vi "Draw.vi"(8 "error in (no error)":errorcluster, 9 "disable contained items?":bool, 10 "IB_SourceTree in":refnum<class "IB_Tree.lvclass">, 11 "IB_TreeMyComputer in":refnum<class "IB_Tree_Item_Proj_MyComputer.lvclass">) -> (0 "error out":errorcluster, 3 "IB_TreeItem out":refnum<class "IB_Tree_Item_Proj_MyComputer.lvclass">)   [LabVIEW 2020, in "IB_Tree_Item_Proj_MyComputer.lvclass"]
uses:
  <vilib>/AppBuilder/IB_Classes/Tree_Item_Proj_MyComputer/IB_Tree_Item_Proj_MyComputer.lvclass
  <vilib>/AppBuilder/IB_Classes/Tree_Item_Proj_MyComputer/IB_Tree_Item_Proj_MyComputer.lvclass/IB_Tree_Item_Proj_MyComputer.ctl
  <resource>/Framework/Providers/Builds/Installer/controls/IB_Tree_DefaultSymbols.ctl
  <vilib>/AppBuilder/IB_Classes/Tree_Source/IB_Tree_Source.lvclass
  <vilib>/AppBuilder/IB_Classes/Tree/IB_Tree.lvclass
  <vilib>/AppBuilder/IB_Classes/Tree_Item/IB_Tree_Item.lvclass
  <vilib>/AppBuilder/IB_Classes/Tree_Item_Proj/IB_Tree_Item_Proj.lvclass
  e:/builds/penguin/labview/branches/2020/dev/dist/vi.lib/AppBuilder/IB_Classes/Tree_Item_Proj_Container/IB_Tree_Item_Proj_Container.lvclass
  e:/builds/penguin/labview/branches/2020/dev/dist/vi.lib/AppBuilder/IB_Classes/Tree_Item_Proj/IB_Tree_Item_Proj.lvclass
  e:/builds/penguin/labview/branches/2020/dev/dist/vi.lib/AppBuilder/IB_Classes/Tree_Item/IB_Tree_Item.lvclass
  e:/builds/penguin/labview/branches/2020/dev/dist/vi.lib/AppBuilder/IB_Classes/Tree_Item_Proj_MyComputer/IB_Tree_Item_Proj_MyComputer.lvclass
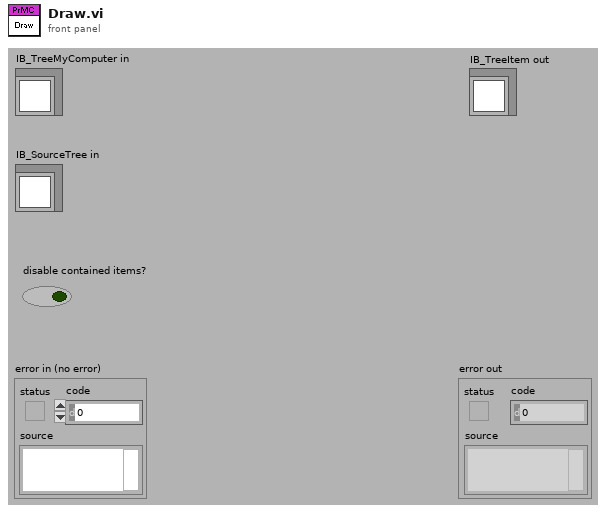
[diagram p1: front panel]
types:
  T1 = typedef "IB_Tree_DefaultSymbols.ctl" = enum16{"<unknown>", "closed folder", "open folder", "closed folder (default)", "open folder (default)", "closed sync folder", "open sync folder", "container folder", "my computer", "build specs", "exe", "dll", "source dist", "restful web service", ".net", "packed library", "c-generator", "target"}
  T2 = typedef "IB_Tree_Source.ctl" = cluster{"buildObject":T3}
  T3 = typedef "ItemRef.ctl" = u64
  T4 = typedef "IB_Tree_Item_Proj.ctl" = cluster{"itemID":string, "path":path}
  T5 = typedef "IB_Tree_Item.ctl" = cluster{"symbol index":i32, "child tag":string, "parentTag":string, "left cell name":string}
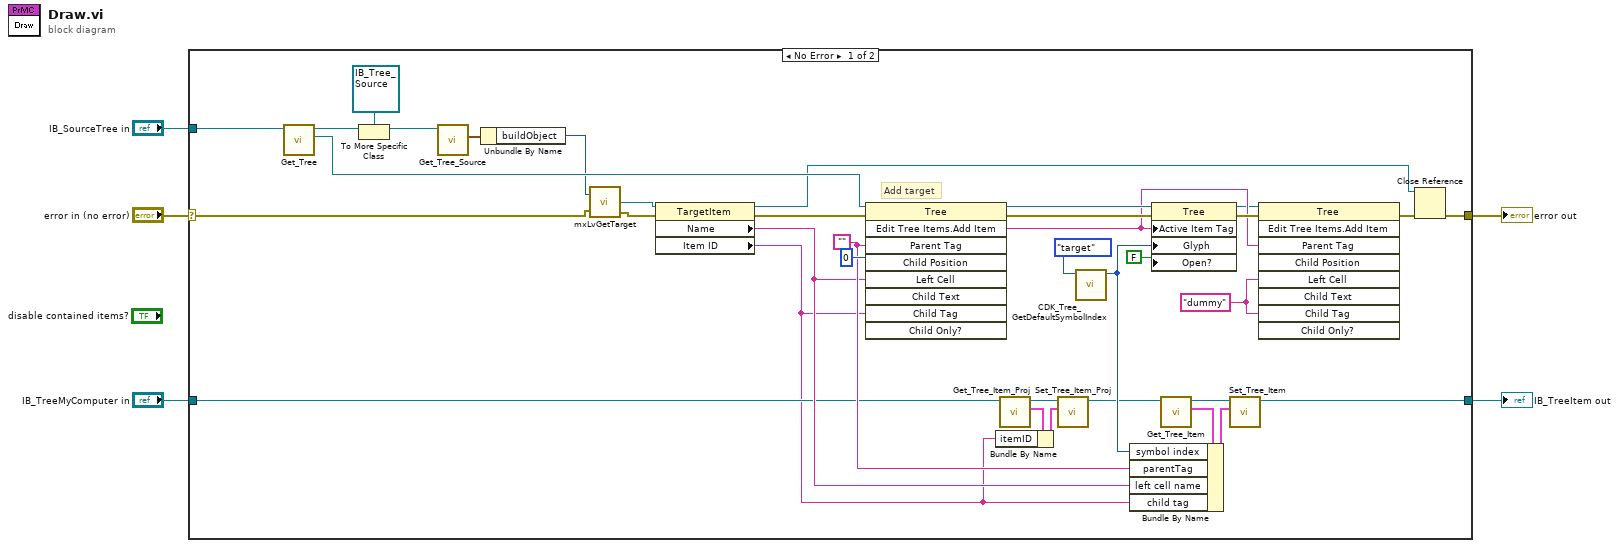
[diagram p0: block diagram]
diagram:
  n1 = case shown="No Error" "error in (no error)" {
    selector: "error in (no error)" -> [w9 w43]
    tunnel: [w18 w43] -> w4
    tunnel: "IB_SourceTree in" -> [w34 _]
    tunnel: [w10 w42] -> w2
    tunnel: "IB_TreeMyComputer in" -> [w13 w42]
    frame No Error {
      w30 = "dummy" ("Left Cell String")
      w22 = ""
      # "Add target"
      n2 = call <vilib>:"Get_Tree.vi"("IB_Tree in"=w34) -> ("ctl"=w33:refnum<vi>, "IB_Tree out"=w27:refnum<class "IB_Tree.lvclass">)  [unwired: 1 in, 8 out]
      n3 = To More Specific Class(target class=refnum<class "IB_Tree_Source.lvclass"> refnum ("IB_SourceTree.lvclass"), reference=w27) -> (specific class reference=w26:refnum<class "IB_Tree_Source.lvclass">)  [unwired: 1 in, 1 out]
      n4 = call <vilib>:"Get_Tree_Source.vi"("IB_SourceTree in"=w26) -> ("data"=w35:T2)  [unwired: 1 in, 9 out]
      n5 = Unbundle By Name(w35) -> ("buildObject"=w6:T3)
      n6 = call <resource>:"mxLvGetTarget.vi"("Item"=w6, "error in"=w9) -> ("Target"=w7:refnum<vi>, "error out"=w8:errorcluster)  [unwired: 1 out]
      n7 = property class="TargetItem"(reference=w7, error in=w8) -> (reference out=w19:refnum<vi>, error out=w38:errorcluster, "Name"=w21:string, "Item ID"=w11:string)
      n8 = invoke class="Tree" method="Edit Tree Items.Add Item"(reference=w33, error in=w38, "Parent Tag"=w22, "Child Position"=0, "Left Cell"=w21, "Child Tag"=w11) -> (reference out=w40:refnum<vi>, error out=w36:errorcluster, "Edit Tree Items:Add Item"=w31:string)  [unwired: 3 in, 6 out]
      n9 = call <vilib>:"Get_Tree_Item_Proj.vi"("IB_TreeProjectItem in"=w13) -> ("data"=w15:T4, "IB_TreeProjectItem out"=w16:refnum<class "IB_Tree_Item_Proj_MyComputer.lvclass">)  [unwired: 1 in, 8 out]
      n10 = Bundle By Name(cluster=w15, "itemID"=w11) -> (w14:T4)
      n11 = call <vilib>:"Set_Tree_Item_Proj.vi"("data"=w14, "IB_TreeProjectItem in"=w16) -> ("IB_TreeProjectItem out"=w12:refnum<class "IB_Tree_Item_Proj_MyComputer.lvclass">)  [unwired: 1 in, 8 out]
      n12 = call <resource>:"CDK_Tree_GetDefaultSymbolIndex.vi"("default symbol"=IB_Tree_DefaultSymbols."target") -> ("symbol index"=w17:i32)  [unwired: 1 in, 9 out]
      n13 = property class="Tree"(reference=w40, error in=w36, "Active Item Tag"=w31, "Glyph"=w17, "Open?"=FALSE ("Active Item:Open?")) -> (reference out=w29:refnum<vi>, error out=w32:errorcluster)
      n14 = call <vilib>:"Get_Tree_Item.vi"("IB_TreeItem in"=w12) -> ("data"=w24:T5, "IB_TreeItem out"=w25:refnum<class "IB_Tree_Item_Proj_MyComputer.lvclass">)  [unwired: 1 in, 8 out]
      n15 = Bundle By Name(cluster=w24, "symbol index"=w17, "parentTag"=w22, "left cell name"=w21, "child tag"=w11) -> (w23:T5)
      n16 = call <vilib>:"Set_Tree_Item.vi"("data"=w23, "IB_TreeItem in"=w25) -> ("IB_TreeItem out"=w10:refnum<class "IB_Tree_Item_Proj_MyComputer.lvclass">)  [unwired: 1 in, 8 out]
      n17 = invoke class="Tree" method="Edit Tree Items.Add Item"(reference=w29, error in=w32, "Parent Tag"=w31, "Left Cell"=w30, "Child Tag"=w30) -> (error out=w20:errorcluster)  [unwired: 4 in, 8 out]
      n18 = Close Reference(reference=w19, error in (no error)=w20) -> (error out=w18:errorcluster)
    }
    frame Error {
    }
  }
  "error out" <- w4
  "IB_TreeItem out" <- w2
